vi "S-parameters Graph.vi"() -> ()   [LabVIEW 2023, in "NI_HFNetworkAnalysis.lvlib"]
uses:
  NI_HFNetworkAnalysis.lvlib
panel:
  in  "S-par":u16(ring) items=["S11", "S21", "S12", "S22"]
  in  "Format":u16(ring) items=["Ampl (dB)", "Ampl (mag)", "Phase (deg)", "Phase (rad)", "Re", "Im"]
  out "S-parameter Graph":T1(graph)
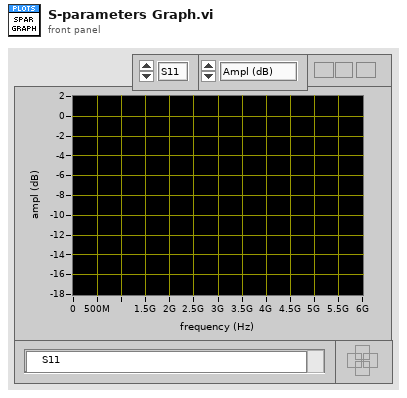
[diagram p1: front panel]
types:
  T1 = cluster{"FrequencyList":dbl[], "Array out":dbl[]}
  T2 = cluster{"Frequencies":dbl[], "Formatted S-parameter":dbl[]}
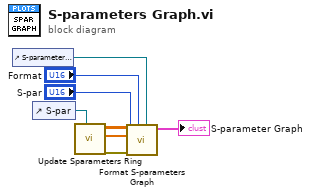
[diagram p0: block diagram]
diagram:
  n1 = control-ref of="S-parameter Graph"() -> (w7:refnum<vi>)
  n2 = control-ref of="S-par"() -> (w1:refnum<vi>)
  n3 = call "Update Sparameters Ring.vi"("S-par reference"=w1) -> ("error out"=w6:errorcluster, "Frequencies out"=w4:dbl[], "S-parameters out"=w5:cdb[][])  [unwired: 7 in, 1 out]
  n4 = call "Format S-parameters Graph.vi"("S-parameter reference"=w7, "Format"="Format", "error in (no error)"=w6, "S-parameter Index"="S-par", "Frequencies"=w4, "S-parameters"=w5) -> ("S-parameter Graph"=→"S-parameter Graph":T2)  [unwired: 4 in, 1 out]
